vi "Get Path.vi"(11 "jettl Actor in":refnum<class "jettl Actor.lvclass">) -> (2 "Path":path)   [LabVIEW 2021, in "jettl.lvlib" / "Temporary Actor.lvlib" / "jettl Actor.lvclass"]
uses:
  jettl Actor.lvclass
  jettl Actor.lvclass/jettl Actor.ctl
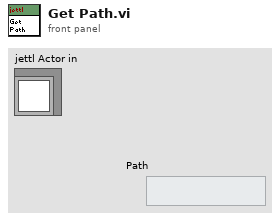
[diagram p1: front panel]
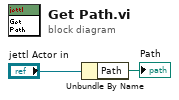
[diagram p0: block diagram]
diagram:
  n1 = Unbundle By Name("jettl Actor in") -> ("Path"=→"Path":path)
